vi "algo.search.is.final.vi"(8 "buy":bool, 9 "isLast":bool, 10 "isFirst":bool, 11 "Direction":i8=-1) -> (3 "isFinal":bool)   [LabVIEW 2022 SP3]
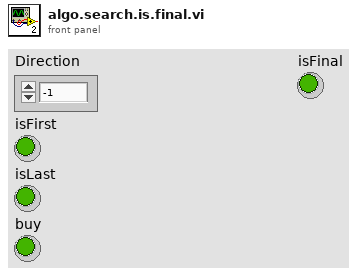
[diagram p1: front panel]
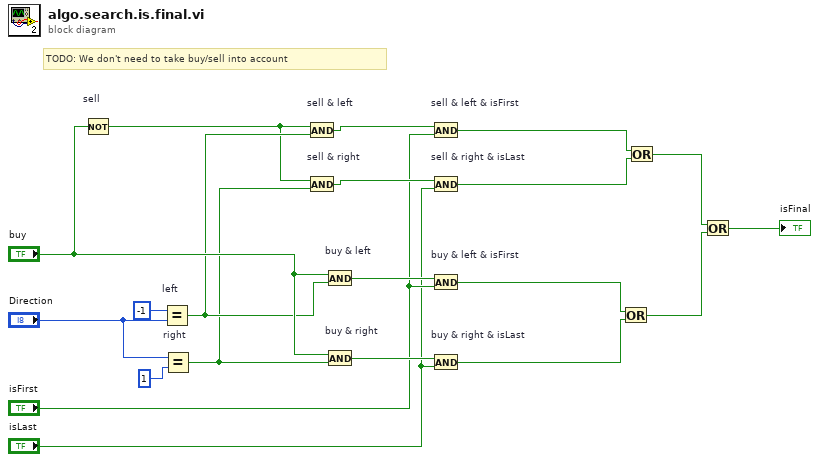
[diagram p0: block diagram]
diagram:
  # "TODO: We don't need to take buy/sell into account"
  n1 = Not "sell"(x="buy") -> (.not. x?=w13:bool)
  n2 = Equal? "left"(x=i8 -1, y="Direction") -> (x = y?=w14:bool)
  n3 = Equal? "right"(x="Direction", y=i8 1 ("x")) -> (x = y?=w12:bool)
  n4 = And "sell & left"(x=w13, y=w14) -> (x .and. y?=w11:bool)
  n5 = And "sell & right"(x=w13, y=w12) -> (x .and. y?=w10:bool)
  n6 = And "buy & left"(x="buy", y=w14) -> (x .and. y?=w17:bool)
  n7 = And "buy & right"(x="buy", y=w12) -> (x .and. y?=w15:bool)
  n8 = And "sell & left & isFirst"(x=w11, y="isFirst") -> (x .and. y?=w6:bool)
  n9 = And "sell & right & isLast"(x=w10, y="isLast") -> (x .and. y?=w7:bool)
  n10 = And "buy & left & isFirst"(x=w17, y="isFirst") -> (x .and. y?=w8:bool)
  n11 = And "buy & right & isLast"(x=w15, y="isLast") -> (x .and. y?=w9:bool)
  n12 = Or(x=w8, y=w9) -> (x .or. y?=w4:bool)
  n13 = Or(x=w6, y=w7) -> (x .or. y?=w5:bool)
  n14 = Or(x=w5, y=w4) -> (x .or. y?=→"isFinal":bool)
